vi "Read Section Delimiter.vi"(11 "ConfigManager.Text in":refnum<class "ConfigManager.Text.lvclass">) -> (2 "Section Delimiter":refnum<class "Delimiter.lvclass">, 3 "ConfigManager.Text out":refnum<class "ConfigManager.Text.lvclass">)   [LabVIEW 2013, in "CfgManager.Text.lvlib" / "ConfigManager.Text.lvclass"]
uses:
  ConfigManager.Text.lvclass
  <vilib>/LabVIEW Open Source Project/Unicity/Delimiter/Delimiter.lvclass
  ConfigManager.Text.lvclass/ConfigManager.Text.ctl
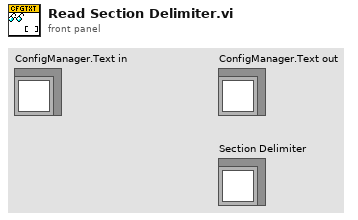
[diagram p1: front panel]
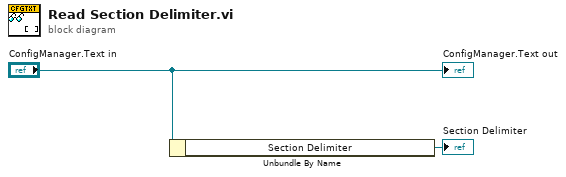
[diagram p0: block diagram]
diagram:
  n1 = Unbundle By Name("ConfigManager.Text in") -> ("Section Delimiter"=→"Section Delimiter":refnum<class "Delimiter.lvclass">)
  "ConfigManager.Text out" <- "ConfigManager.Text in"
